vi "Event_Exam.vi"() -> ()   [LabVIEW 2018]
panel:
  out "구구단":string[][](array[string])
  in  "실행 버튼":bool
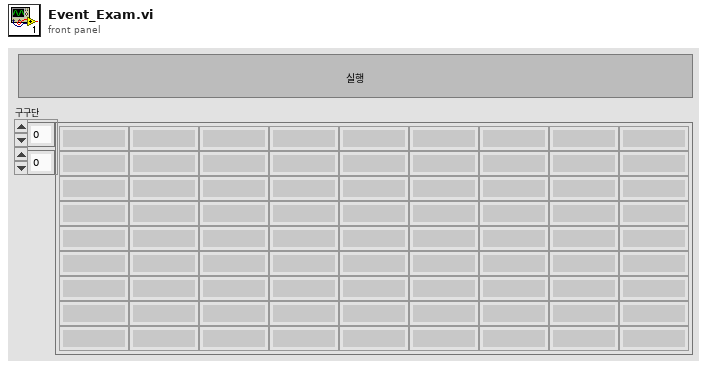
[diagram p1: front panel]
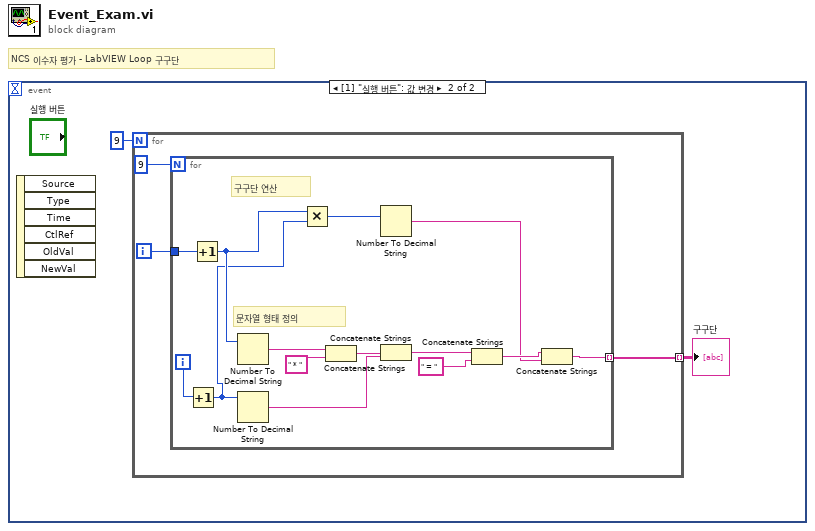
[diagram p0: block diagram]
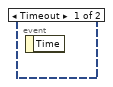
[diagram p2: hidden frame]
diagram:
  # "NCS 이수자 평가 - LabVIEW Loop 구구단"
  n1 = event shown="[1] \"실행 버튼\": 값 변경" {
    selector: _ -> [_ _]
    dyn-events: _ -> [_ _]
    timeout: _ -> [_ _]
    event Timeout {
      n2 = event-data() -> ()  [unwired: 1 in, 1 out]
    }
    event "실행 버튼": Value Change {
      n3 = event-data() -> ()  [unwired: 1 in, 6 out]
      n4 = for {
        N: 9 -> [_]
        tunnel: [w3] -> w1 mode=indexing
        i -> [w4]
        n5 = for {
          N: 9 -> [_]
          tunnel: w4 -> [w12]
          tunnel: [w6] -> w3 mode=indexing
          i -> [w13]
          # "문자열 형태 정의"
          # "구구단 연산"
          n6 = Increment(x=w13) -> (x+1=w10:i32)
          n7 = Increment(x=w12) -> (x+1=w11:i32)
          n8 = Number To Decimal String(number=w11) -> (decimal integer string=w19:string)  [unwired: 1 in]
          n9 = Number To Decimal String(number=w10) -> (decimal integer string=w16:string)  [unwired: 1 in]
          n10 = Multiply(x=w11, y=w10) -> (x*y=w8:i32)
          n11 = Concatenate Strings(w19, " * ") -> (w17:string)
          n12 = Number To Decimal String(number=w8) -> (decimal integer string=w7:string)  [unwired: 1 in]
          n13 = Concatenate Strings(w17, w16) -> (w15:string)
          n14 = Concatenate Strings(w15, " = ") -> (w9:string)
          n15 = Concatenate Strings(w9, w7) -> (w6:string)
        }
      }
      "구구단" <- w1
    }
  }
